vi "Init.vi"(8 "error in (no error)":errorcluster, 11 "SLMP in":refnum<class "SLMP.lvclass">) -> (0 "error out":errorcluster, 3 "SLMP out":refnum<class "SLMP.lvclass">)   [LabVIEW 2019, in "SLMP.lvlib" / "SLMP.lvclass"]
uses:
  SLMP.lvclass
  SLMP.lvclass/SLMP.ctl
  SLMP.lvlib
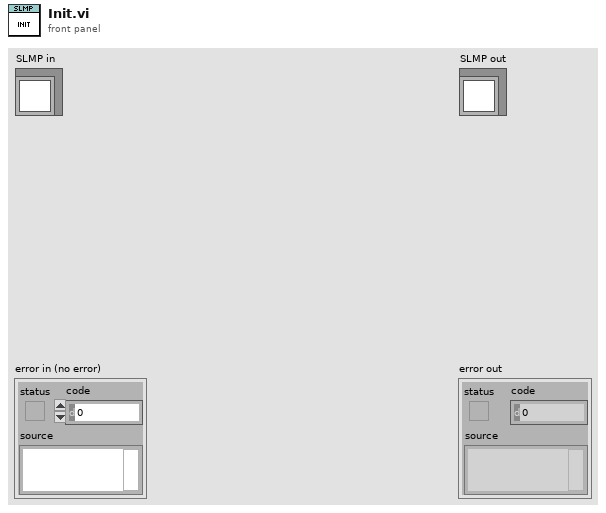
[diagram p1: front panel]
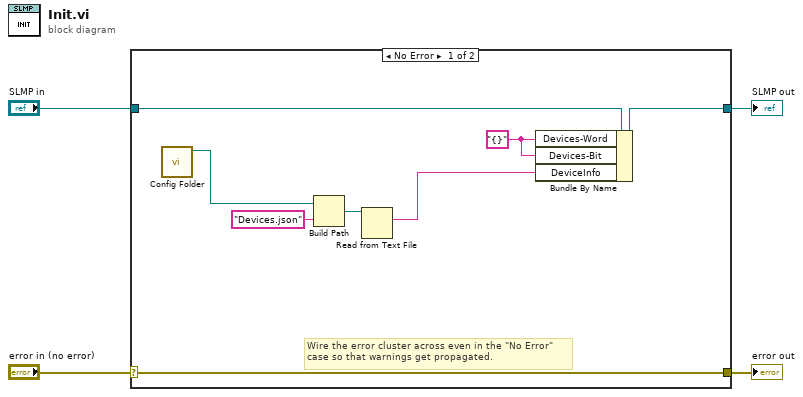
[diagram p0: block diagram]
diagram:
  n1 = case shown="No Error" "error in (no error)" {
    selector: "error in (no error)" -> [w11 w14]
    tunnel: [w11 w14] -> w3
    tunnel: [w7 w13] -> w1
    tunnel: "SLMP in" -> [w12 w13]
    frame No Error {
      w5 = "{}"
      # "Wire the error cluster across even in the \"No Error\"\ncase so that warnings get propagated."
      n2 = call "Config Folder.vi"() -> (".config folder"=w10:path)  [unwired: 11 in]
      n3 = Build Path(base path=w10, name or relative path="Devices.json") -> (appended path=w8:path)
      n4 = Read from Text File(file (use dialog)=w8) -> (text=w6:string)  [unwired: 3 in, 3 out]
      n5 = Bundle By Name(cluster=w12, "Devices-Word"=w5, "Devices-Bit"=w5, "DeviceInfo"=w6) -> (w7:refnum<class "SLMP.lvclass">)
    }
    frame Error {
    }
  }
  "error out" <- w3
  "SLMP out" <- w1
